vi "SPI Read Bytes Of Event.vi"(4 "TimeOutOfMs":i32, 5 "EventType":u8, 6 "EventPin":i32, 7 "ReadLen":i32, 9 "pReadData":u8[](array[numeric])=array[4097 elements], 10 "SPIIndex":i32, 11 "DevHandle":i32) -> (1 "pReadData out":u8[](array[numeric]), 3 "function return":i32)   [LabVIEW 2010, in "usb2spi.lvlib"]
doc: "int WINAPI SPI_ReadBytesOfEvent(int DevHandle,int SPIIndex,unsigned char *pReadData,int ReadLen,int EventPin,unsigned char EventType,int TimeOutOfMs);"
uses:
  usb2spi.lvlib
  USB2XXX/trunk/USB2XXX/USB2XXX/vs2019/Release/USB2XXX.dll
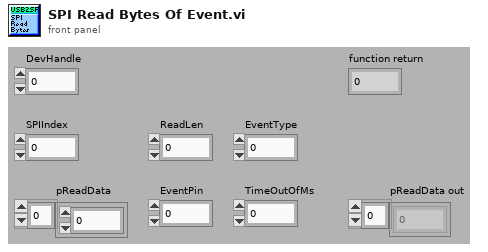
[diagram p1: front panel]
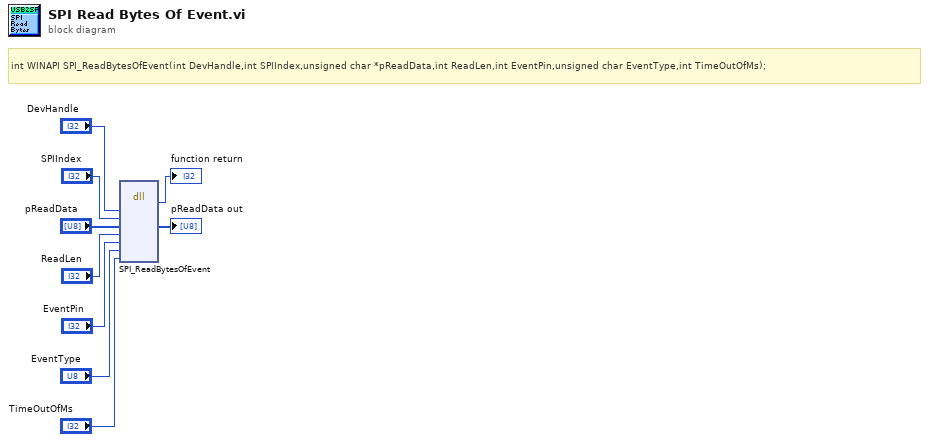
[diagram p0: block diagram]
diagram:
  # "int WINAPI SPI_ReadBytesOfEvent(int DevHandle,int SPIIndex,unsigned char *pReadData,int ReadLen,int EventPin,unsigned char EventType,int TimeOutOfMs);"
  n1 = dll-call lib="E:/Projects/USB2XXX/trunk/USB2XXX/USB2XXX/vs2019/Release/USB2XXX.*" fn="SPI_ReadBytesOfEvent"("DevHandle"="DevHandle", "SPIIndex"="SPIIndex", "pReadData"="pReadData", "ReadLen"="ReadLen", "EventPin"="EventPin", "EventType"="EventType", "TimeOutOfMs"="TimeOutOfMs") -> (→"function return":i32, "pReadData"=→"pReadData out":u8[])  [unwired: 9 in, 2 out]
